vi "AlliGator Calibration Frequency Dialog.vi"(1 "Calibration Phasor Frequency":dbl[unit], 2 "Internal Phasor Frequency":dbl[unit]) -> (0 "Use Calibration Frequency?":bool)   [LabVIEW 2021, in "AlliGator Phasor Calibration.lvlib"]
doc: "Dialog opened when the phasor frequency stored in a calibration file is different from the current one.\n\nOffers to ignore the file, or load it and replace the current phasor frequency with that stored in the file."
uses:
  AlliGator Phasor Calibration.lvlib
panel:
  in  "Keep":bool
  in  "Replace":bool
  out "Message":string
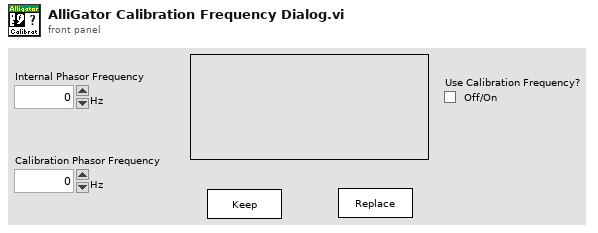
[diagram p1: front panel]
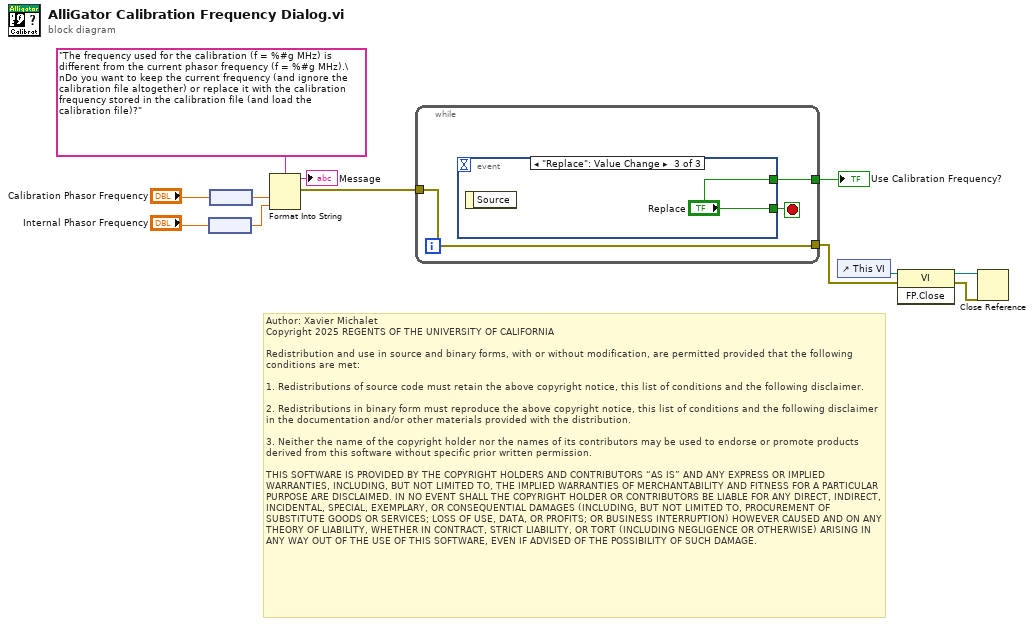
[diagram p0: block diagram]
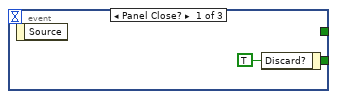
[diagram p2: hidden frame]
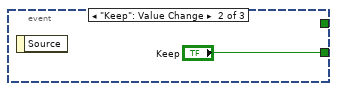
[diagram p3: hidden frame]
diagram:
  # "Author: Xavier Michalet\nCopyright 2025 REGENTS OF THE UNIVERSITY OF CALIFORNIA\n\nRedistribution and use in source and binary forms, with or without modification, are permitted provided that the following conditions are met:\n\n1. Redistributions of source code must retain the above copyright notice, this list of conditions and the following disclaimer.\n\n2. Redistributions in binary form must reproduce the above copyright notice, this list of conditions and the following disclaimer in the documentation and/or other materials provided with the distribution.\n\n3. Neither the name of the copyright holder nor the names of its contributors may be used to endorse or promote products derived from this software without specific prior written permission.\n\nTHIS SOFTWARE IS PROVIDED BY THE COPYRIGHT HOLDERS AND CONTRIBUTORS “AS IS” AND ANY EXPRESS OR IMPLIED WARRANTIES, INCLUDING, BUT NOT LIMITED TO, THE IMPLIED WARRANTIES OF MERCHANTABILITY AND FITNESS FOR A PARTICULAR PURPOSE ARE DISCLAIMED. IN NO EVENT SHALL THE COPYRIGHT HOLDER OR CONTRIBUTORS BE LIABLE FOR ANY DIRECT, INDIRECT, INCIDENTAL, SPECIAL, EXEMPLARY, OR CONSEQUENTIAL DAMAGES (INCLUDING, BUT NOT LIMITED TO, PROCUREMENT OF SUBSTITUTE GOODS OR SERVICES; LOSS OF USE, DATA, OR PROFITS; OR BUSINESS INTERRUPTION) HOWEVER CAUSED AND ON ANY THEORY OF LIABILITY, WHETHER IN CONTRACT, STRICT LIABILITY, OR TORT (INCLUDING NEGLIGENCE OR OTHERWISE) ARISING IN ANY WAY OUT OF THE USE OF THIS SOFTWARE, EVEN IF ADVISED OF THE POSSIBILITY OF SUCH DAMAGE."
  n1 = node("Internal Phasor Frequency") -> (w8:dbl)
  n2 = node("Calibration Phasor Frequency") -> (w10:dbl)
  n3 = Format Into String(format string="The frequency used for the calibration (f = %#g MHz) is different from the current phasor frequency (f = %#g MHz).\nDo you want to keep the current frequency (and ignore the calibration file altogether) or replace it with the calibration frequency stored in the calibration file (and load the calibration file)?", w10, w8) -> (resulting string=→"Message":string, error out=w6:errorcluster)  [unwired: 2 in]
  n4 = while {
    tunnel: w6 -> [w13]
    tunnel: [w14] -> w5
    tunnel: [w13] -> w4
    stop <- w15 stop-if-true
    n5 = event shown="[2] \"Replace\": Value Change" {
      selector: _ -> [_ _ _]
      dyn-events: _ -> [_ _ _]
      timeout: _ -> [_ _ _]
      tunnel: [w16 "Keep" "Replace"] -> w15
      tunnel: [_ _ "Replace"] -> w14
      event Panel Close? {
        w16 = TRUE ("Discard?")
        n6 = event-data() -> ()  [unwired: 1 in, 1 out]
        n7 = event-data("Discard?"=w16) -> ()  [unwired: 1 in, 1 out]
      }
      event "Keep": Value Change {
        n8 = event-data() -> ()  [unwired: 1 in, 1 out]
      }
      event "Replace": Value Change {
        n9 = event-data() -> ()  [unwired: 1 in, 1 out]
      }
    }
  }
  "Use Calibration Frequency?" <- w5
  n10 = control-ref of="This VI"() -> (w3:refnum<vi>)
  n11 = invoke class="VI" method="FP.Close"(reference=w3, error in=w4) -> (reference out=w2:refnum<vi>, error out=w1:errorcluster)  [unwired: 1 in, 1 out]
  n12 = Close Reference(reference=w2, error in (no error)=w1) -> ()  [unwired: 1 out]
